vi "niWLAN - 80211abgnRxMeasurementsRW.vi"(0 "Array":T1(array[cluster]), 1 "file path (dialog if empty)":path, 5 "Rx Measurements Settings":T2 {"DSSS Data Rate (Mbps)" items=["1", "2", "5.5 CCK", "5.5 PBCC", "11 CCK", "11 PBCC", "22", "33"]; "OFDM Data Rate (Mbps)" items=["6", "9", "12", "18", "24", "36", "48", "54"]; "80211n PLCP Frame Format" items=["Mixed Format", "Greenfield Format"]; "Standard" items=["80211A/G/J/P OFDM", "80211B/G DSSS", "80211G DSSSOFDM", "80211N MIMOOFDM", "80211AC MIMOOFDM"]}, 11 "error in (no error)":errorcluster) -> ()   [LabVIEW 2011]
uses:
  TV/RW/Includes/WLAN - TV - RW - INC - TV_Format_Rx.ctl
  <vilib>/Utility/file.llb/Write To Spreadsheet File (string).vi
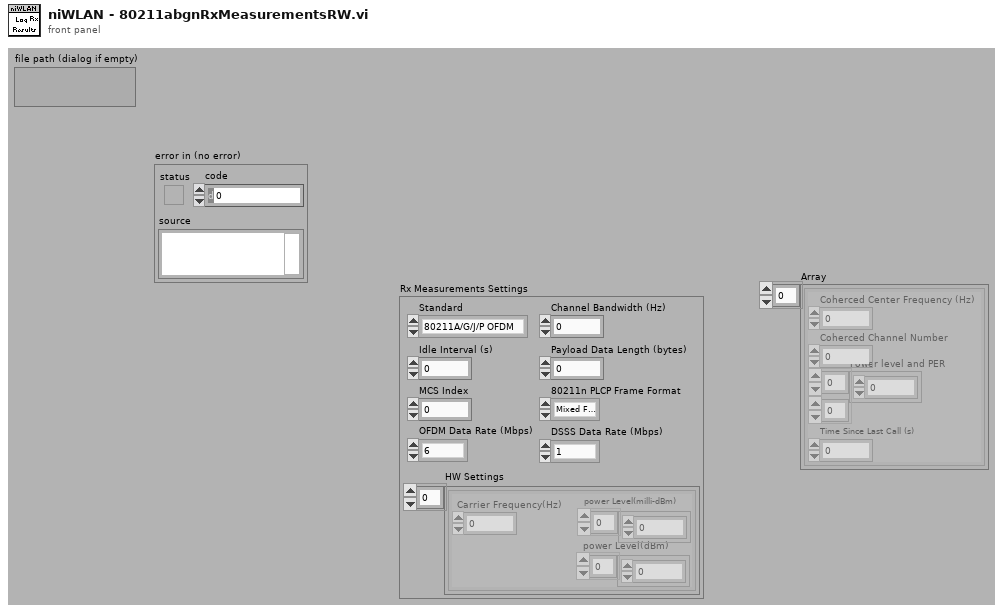
[diagram p1: front panel]
types:
  T1 = cluster{"Coherced Center Frequency (Hz)":dbl, "Coherced Channel Number":i32, "Power level and PER":dbl[][], "Time Since Last Call (s)":dbl}[]
  T2 = typedef "WLAN - TV - RW - INC - TV_Format_Rx.ctl" = cluster{"Standard":i32, "Channel Bandwidth (Hz)":dbl, "Idle Interval (s)":dbl, "MCS Index":i32, "80211n PLCP Frame Format":i32, "Payload Data Length (bytes)":i32, "OFDM Data Rate (Mbps)":i32, "DSSS Data Rate (Mbps)":i32, "HW Settings":cluster{"Carrier Frequency(Hz)":dbl, "power Level(dBm)":dbl[], "power Level(milli-dBm)":i32[]}[]}
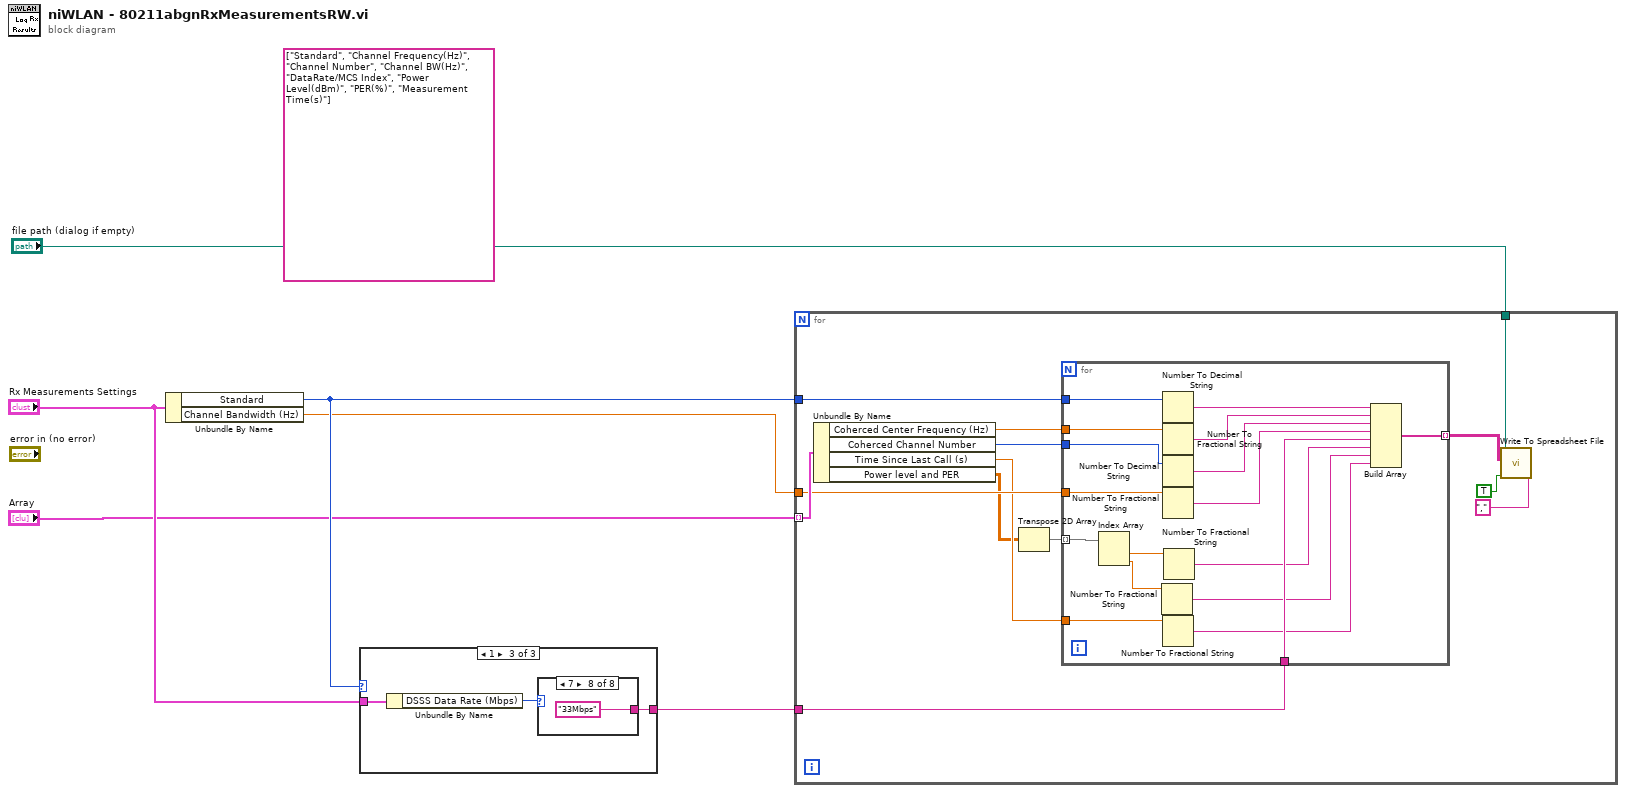
[diagram p0: block diagram]
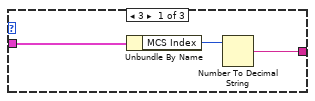
[diagram p2: hidden frame]
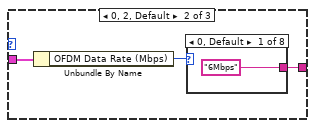
[diagram p3: hidden frame]
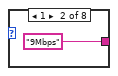
[diagram p4: hidden frame]
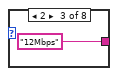
[diagram p5: hidden frame]
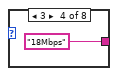
[diagram p6: hidden frame]
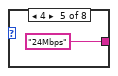
[diagram p7: hidden frame]
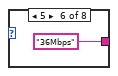
[diagram p8: hidden frame]
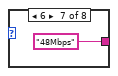
[diagram p9: hidden frame]
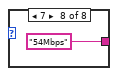
[diagram p10: hidden frame]
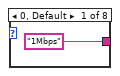
[diagram p11: hidden frame]
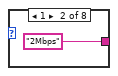
[diagram p12: hidden frame]
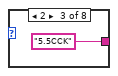
[diagram p13: hidden frame]
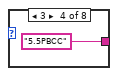
[diagram p14: hidden frame]
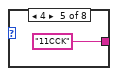
[diagram p15: hidden frame]
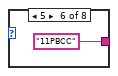
[diagram p16: hidden frame]
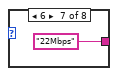
[diagram p17: hidden frame]
diagram:
  (unwired) string[] ["Standard", "Channel Frequency(Hz)", "Channel Number", "Channel BW(Hz)", "DataRate/MCS Index", "Power Level(dBm)", "PER(%)", "Measurement Time(s)"]
  n1 = Unbundle By Name("Rx Measurements Settings") -> ("Standard"=w5:i32, "Channel Bandwidth (Hz)"=w2:dbl)
  n2 = case shown="1" w5 {
    tunnel: "Rx Measurements Settings" -> [w9 w12 w23]
    tunnel: [w7 w10 w21] -> w6
    frame 3 {
      n3 = Unbundle By Name(w9) -> ("MCS Index"=w8:i32)
      n4 = Number To Decimal String(number=w8) -> (decimal integer string=w7:string)  [unwired: 1 in]
    }
    frame 0, 2, Default {
      n5 = Unbundle By Name(w12) -> ("OFDM Data Rate (Mbps)"=w11:i32)
      n6 = case shown="0, Default" w11 {
        tunnel: ["6Mbps" ("active channel") "9Mbps" ("active channel") "12Mbps" ("active channel") "18Mbps" ("active channel") "24Mbps" ("active channel") "36Mbps" ("active channel") "48Mbps" ("active channel") "54Mbps" ("active channel")] -> w10
        frame 0, Default {
        }
        frame 1 {
        }
        frame 2 {
        }
        frame 3 {
        }
        frame 4 {
        }
        frame 5 {
        }
        frame 6 {
        }
        frame 7 {
        }
      }
    }
    frame 1 {
      n7 = Unbundle By Name(w23) -> ("DSSS Data Rate (Mbps)"=w22:i32)
      n8 = case shown="7" w22 {
        tunnel: ["1Mbps" ("active channel") "2Mbps" ("active channel") "5.5CCK" ("active channel") "5.5PBCC" ("active channel") "11CCK" ("active channel") "11PBCC" ("active channel") "22Mbps" ("active channel") "33Mbps" ("active channel")] -> w21
        frame 0, Default {
        }
        frame 1 {
        }
        frame 2 {
        }
        frame 3 {
        }
        frame 4 {
        }
        frame 5 {
        }
        frame 6 {
        }
        frame 7 {
        }
      }
    }
  }
  n9 = for {
    tunnel: w6 -> [w44]
    tunnel: w5 -> [w43]
    tunnel: "Array" -> [w42] mode=indexing
    tunnel: w2 -> [w39]
    tunnel: "file path (dialog if empty)" -> [w35]
    n10 = Unbundle By Name(w42) -> ("Coherced Center Frequency (Hz)"=w41:dbl, "Coherced Channel Number"=w40:i32, "Time Since Last Call (s)"=w38:dbl, "Power level and PER"=w34:dbl[][])
    n11 = Transpose 2D Array(2D array=w34) -> (transposed array=w33:dbl[][])
    n12 = for {
      tunnel: w44 -> [w57]
      tunnel: w43 -> [w54]
      tunnel: w41 -> [w53]
      tunnel: w40 -> [w52]
      tunnel: w39 -> [w51]
      tunnel: w38 -> [w50]
      tunnel: w33 -> [w49] mode=indexing
      tunnel: [w45] -> w32 mode=indexing
      n13 = Index Array(array=w49) -> (element #1=w48:dbl, element #2=w46:dbl)  [unwired: 2 in]
      n14 = Number To Fractional String(number=w46) -> (F-format string=w47:string)  [unwired: 3 in]
      n15 = Number To Decimal String(number=w54) -> (decimal integer string=w61:string)  [unwired: 1 in]
      n16 = Number To Fractional String(number=w53) -> (F-format string=w60:string)  [unwired: 3 in]
      n17 = Number To Decimal String(number=w52) -> (decimal integer string=w59:string)  [unwired: 1 in]
      n18 = Number To Fractional String(number=w51) -> (F-format string=w58:string)  [unwired: 3 in]
      n19 = Number To Fractional String(number=w50) -> (F-format string=w55:string)  [unwired: 3 in]
      n20 = Number To Fractional String(number=w48) -> (F-format string=w56:string)  [unwired: 3 in]
      n21 = Build Array(w61, w60, w59, w58, w57, w56, w47, w55) -> (w45:string[])
    }
    n22 = call-poly <vilib>:"Write To Spreadsheet File.vi"("delimiter (\\t)"="," ("delimiter (\\t)"), "append to file? (new file:F)"=TRUE, "2D data"=w32, "file path (dialog if empty)"=w35) -> ()  [unwired: 4 in, 1 out]
  }
